vi "santec laser sweep and oscilloscope.vi"() -> ()   [LabVIEW 2011]
uses:
  <vilib>/Instr/_visa.llb/VISA Open Access Mode.ctl
  <instrlib>/santec TSL/santec TSL-510.lvlib
panel:
  in  "Sweep Stop Wavelength (nm)":dbl=1640.0 min=1250.0 max=1690.0 step=0.001 format="%.3g"
  in  "Sweep Start wavelength (nm)":dbl=1480.0 min=1250.0 max=1690.0 step=0.001 format="%.3g"
  in  "Sweep step (nm)":dbl=1.0 min=0.001 max=120.0 format="%.3g"
  in  "Sweep Speed (nm/s)":dbl=100.0 min=1.0 max=100.0 step=0.1 format="%.1f"
  in  "Sweep Mode (1: Continuous One-way)":i32(ring)=1 format="%#_1f" items=["Step One-way", "Continuous One-way", "Step Two-way", "Continuous Two-way"]
  in  "Step dwell time (s)":dbl=1.0 min=0.0 max=999.9 step=0.1 format="%.1g"
  in  "Sweep Delay (s)":dbl min=0.0 max=999.9000244140625 step=0.10000000149011612 format="%.1g"
  in  "Sweep Cycles":i16=1 min=0 max=999 step=1
  out "Success":bool
  in  "Start (T: Execute)":bool=TRUE
  out "error out":errorcluster
  in  "error in (no error)":errorcluster
  out "dup VISA session":refnum<visa-resource-name>
  in  "VISA session":refnum<visa-resource-name>
  in  "Oscilloscope wait time (ms)":u32
  in  "laser wait time (ms)":u32=1100
  in  "Oscilloscope read time (ms)":u32=4000
  out "error out 2":errorcluster
  in  "Oscilloscope VISA GPIB Resource":refnum<visa-resource-name>="GPIB0::7::INSTR"
  # "Reference Value:\nFor 2.2s, 4Msa/s:\nlaser wait time: 1100ms;\noscilloscope read time: 4000ms;\n\nFor 2s, 400Ksa/s;\nlaser wait time: 1000ms \noscilloscope read time: \n\nFor 5s, 5Mpts oscilloscope setting:\nlaser wait time: 2600ms;\nOscilloscope read time: 8000ms;\n\nFor 20s, 10Mpts setting:\nlaser wait time: 10500ms;\nOscilloscope read time: 35000ms;\nf\nFor 50s, 200Ksa/s setting:\nlaser wait time: 25000ms\nOscilloscope read time: 85000ms;\nChannel offset:\nCH1:\nCH2:\nCH3:\nCH4:"
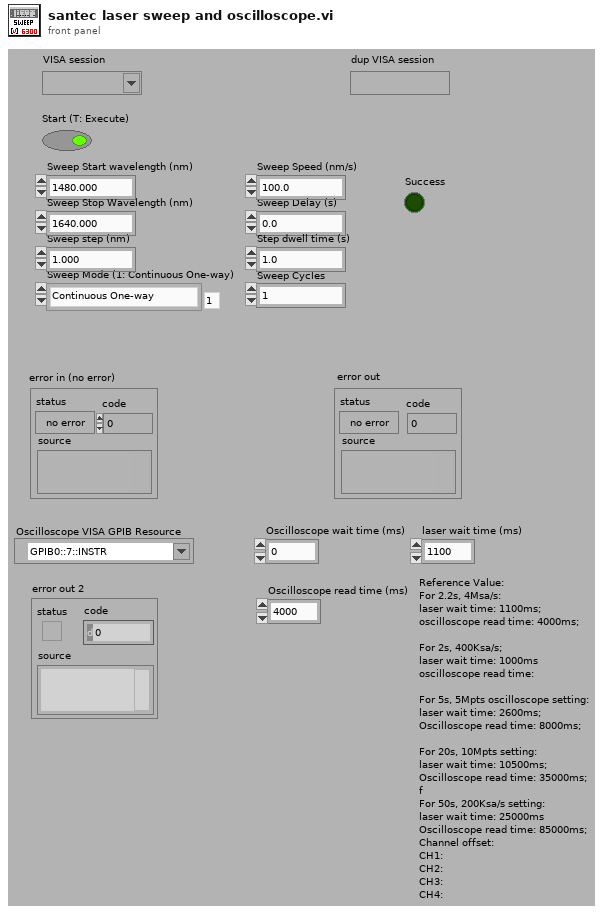
[diagram p1: front panel]
types:
  T1 = enum16{"Identification Query", "Operation Complete Query"}
  T2 = typedef "VISA Open Access Mode.ctl" = u32
  T3 = enum16{"Scan Reset", "Scan Start", "Scan Stop", "Laser On", "Laser Off", "Laser State?", "Track Off"}
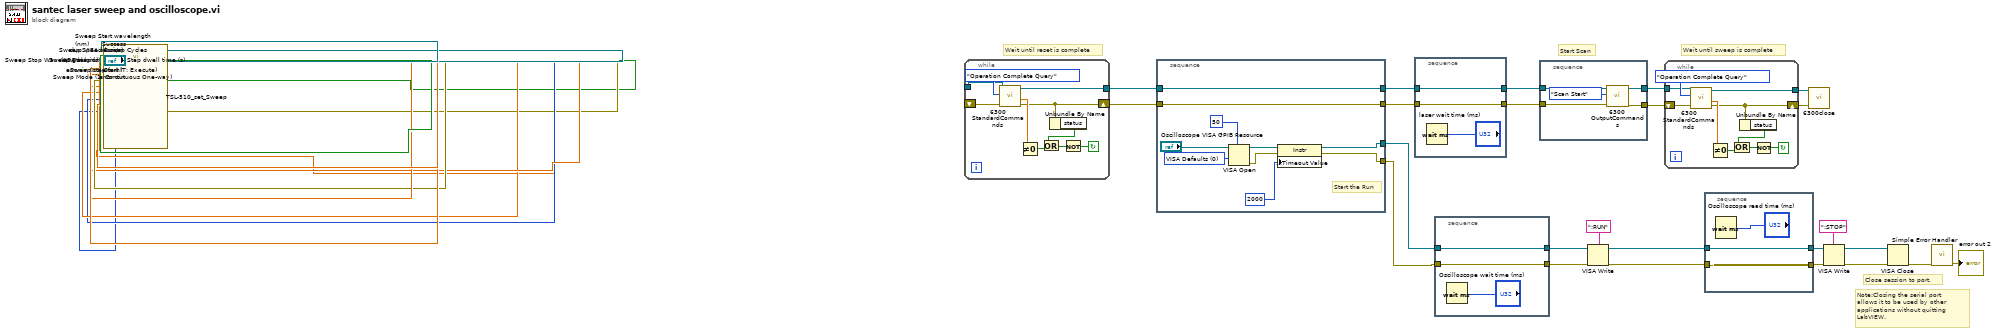
[diagram p0: block diagram]
diagram:
  # "Note:Closing the serial port allows it to be used by other applications without quitting LabVIEW."
  # "Close session to port."
  # "Wait until sweep is complete"
  # "Start Scan"
  # "Wait until reset is complete"
  n1 = call <instrlib>:"TSL-510_set_Sweep.vi"("VISA session"="VISA session", "Start (T: Execute)"="Start (T: Execute)", "Sweep Start wavelength (nm)"="Sweep Start wavelength (nm)", "Sweep Stop Wavelength (nm)"="Sweep Stop Wavelength (nm)", "Sweep step (nm)"="Sweep step (nm)", "error in (no error)"="error in (no error)", "Sweep Mode (1: Continuous One-way)"="Sweep Mode (1: Continuous One-way)", "Sweep Speed (nm/s)"="Sweep Speed (nm/s)", "Sweep Delay (s)"="Sweep Delay (s)", "Step dwell time (s)"="Step dwell time (s)", "Sweep Cycles"="Sweep Cycles") -> ("dup VISA session"=→"dup VISA session":refnum<visa-resource-name>, "Success"=→"Success":bool, "error out"=→"error out":errorcluster)  [unwired: 6 in]
  n2 = while {
    tunnel: [w41] -> w27
    tunnel: _ -> [w45]
    shift-left: _ -> [w44]
    shift-right: [w40] -> w26
    stop <- w43 continue-if-true
    n3 = call <instrlib>:"6300 StandardCommands.VI"("error in"=w44, "System Command?"=T1."Operation Complete Query", "VISA session"=w45) -> ("error out"=w40:errorcluster, "Returned Number"=w46:dbl, "dup VISA session"=w41:refnum<visa-resource-name>)  [unwired: 5 in, 1 out]
    n4 = Not Equal To 0?(x=w46) -> (x != 0?=w47:bool)
    n5 = Unbundle By Name(w40) -> ("status"=w39:bool)
    n6 = Or(x=w39, y=w47) -> (x .or. y?=w42:bool)
    n7 = Not(x=w42) -> (.not. x?=w43:bool)
  }
  n8 = stacked-sequence {
    tunnel: w27 -> [w58]
    tunnel: [w58] -> w25
    tunnel: w26 -> [w57]
    tunnel: [w57] -> w23
    tunnel: [w50] -> w21
    tunnel: [w49] -> w20
    frame #0 {
      w56 = T2 0 items=["VISA Defaults"=0, "Exclusive Lock"=1, "Load Configured Settings"=4] ("Access Mode")
      # "Start the Run"
      n9 = VISA Open(timeout (0)=u32 50 ("VISA Open timeout (0)"), access mode=w56, VISA resource name="Oscilloscope VISA GPIB Resource") -> (VISA resource name=w53:refnum<visa-resource-name>, error out=w54:errorcluster)  [unwired: 2 in]
      n10 = property class="Instr"(reference=w53, error in=w54, "General Settings:Timeout Value"=u32 2000) -> (reference out=w50:refnum<visa-resource-name>, error out=w49:errorcluster)
    }
  }
  n11 = stacked-sequence {
    tunnel: w25 -> [w60]
    tunnel: [w60] -> w24
    tunnel: w23 -> [w59]
    tunnel: [w59] -> w22
    frame #0 {
      n12 = Wait (ms)(milliseconds to wait="laser wait time (ms)") -> ()  [unwired: 1 out]
    }
  }
  n13 = stacked-sequence {
    tunnel: w21 -> [w63]
    tunnel: [w63] -> w17
    tunnel: w20 -> [w62]
    tunnel: [w62] -> w18
    frame #0 {
      n14 = Wait (ms)(milliseconds to wait="Oscilloscope wait time (ms)") -> ()  [unwired: 1 out]
    }
  }
  n15 = stacked-sequence {
    tunnel: w24 -> [w69]
    tunnel: w22 -> [w68]
    tunnel: [w66] -> w37
    tunnel: [w65] -> w38
    frame #0 {
      n16 = call <instrlib>:"6300 OutputCommands.VI"("error in"=w68, "Output Command?"=T3."Scan Start", "VISA session"=w69) -> ("error out"=w66:errorcluster, "dup VISA session"=w65:refnum<visa-resource-name>)  [unwired: 3 in, 4 out]
    }
  }
  n17 = VISA Write(VISA resource name=w17, write buffer=":RUN" ("string to write"), error in (no error)=w18) -> (VISA resource name out=w16:refnum<visa-resource-name>, error out=w15:errorcluster)  [unwired: 1 out]
  n18 = while {
    tunnel: [w72] -> w36
    tunnel: w38 -> [w76]
    shift-left: w37 -> [w75]
    shift-right: [w71] -> w35
    stop <- w74 continue-if-true
    n19 = call <instrlib>:"6300 StandardCommands.VI"("error in"=w75, "System Command?"=T1."Operation Complete Query", "VISA session"=w76) -> ("error out"=w71:errorcluster, "Returned Number"=w77:dbl, "dup VISA session"=w72:refnum<visa-resource-name>)  [unwired: 5 in, 1 out]
    n20 = Not Equal To 0?(x=w77) -> (x != 0?=w78:bool)
    n21 = Unbundle By Name(w71) -> ("status"=w70:bool)
    n22 = Or(x=w70, y=w78) -> (x .or. y?=w73:bool)
    n23 = Not(x=w73) -> (.not. x?=w74:bool)
  }
  n24 = stacked-sequence {
    tunnel: w16 -> [w81]
    tunnel: [w81] -> w29
    tunnel: w15 -> [w80]
    tunnel: [w80] -> w28
    frame #0 {
      n25 = Wait (ms)(milliseconds to wait="Oscilloscope read time (ms)") -> ()  [unwired: 1 out]
    }
  }
  n26 = call <instrlib>:"6300close.vi"("error in"=w35, "VISA session"=w36) -> ()  [unwired: 9 in, 1 out]
  n27 = VISA Write(VISA resource name=w29, write buffer=":STOP" ("string to write"), error in (no error)=w28) -> (VISA resource name out=w30:refnum<visa-resource-name>, error out=w31:errorcluster)  [unwired: 1 out]
  n28 = VISA Close(VISA resource name=w30, error in (no error)=w31) -> (error out=w34:errorcluster)
  n29 = call <vilib>:"Simple Error Handler.vi"("error in (no error)"=w34) -> ("error out"=→"error out 2":errorcluster)  [unwired: 1 in, 7 out]
